vi "Set Content Type.vi"(8 "error in (no error)":errorcluster, 10 "Content-Type":string, 11 "Response in":refnum<class "Response.lvclass">) -> (0 "error out":errorcluster, 3 "Response out":refnum<class "Response.lvclass">)   [LabVIEW 2020, in "HTTP Utils.lvlib" / "Response.lvclass"]
uses:
  Response.lvclass
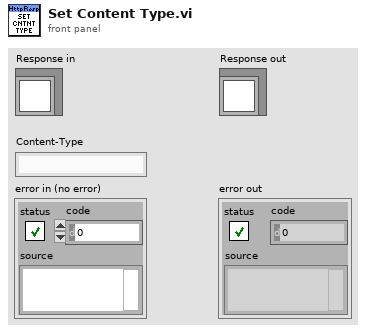
[diagram p1: front panel]
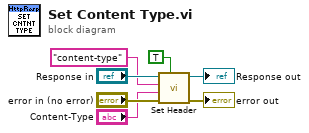
[diagram p0: block diagram]
diagram:
  n1 = call "Set Header.vi"("Replaced Existing (T)"=TRUE, "error in (no error)"="error in (no error)", "Value"="Content-Type", "Header"="content-type", "Response in"="Response in") -> ("error out"=→"error out":errorcluster, "Response out"=→"Response out":refnum<class "Response.lvclass">)  [unwired: 4 in, 1 out]
